vi "Read UI Configuration.vi"(8 "error in":errorcluster, 11 "Bus in":refnum<class "Bus.lvclass">) -> (0 "error out":errorcluster, 2 "UI Configuration":T1, 3 "Bus out":refnum<class "Bus.lvclass">)   [LabVIEW 2014, in "Bus.lvclass"]
uses:
  Bus.lvclass
  UI Configuration.ctl
  Bus Configuration/SPI Configuration.ctl
  Bus.lvclass/Bus.ctl
  Bus Configuration/Bus Configuration.lvclass/Bus Configuration.ctl
  <vilib>/NI/Configuration Framework/serializable configuration/NISE_CEF_serializable configuration.lvclass
  Bus Configuration/Bus Configuration.lvclass
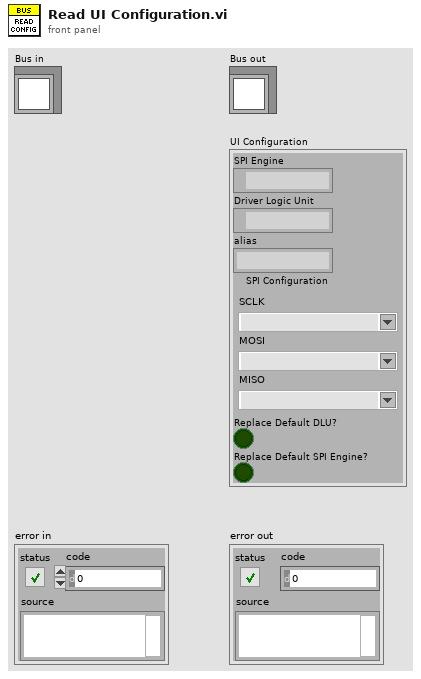
[diagram p1: front panel]
types:
  T1 = typedef "Bus.lvclass/UI Configuration.ctl" = cluster{"SPI Engine":path, "Driver Logic Unit":path, "alias":string, "SPI Configuration":T2, "Replace Default DLU?":bool, "Replace Default SPI Engine?":bool}
  T2 = typedef "Bus Configuration.lvclass/SPI Configuration.ctl" = cluster{"SCLK":string, "MOSI":string, "MISO":string}
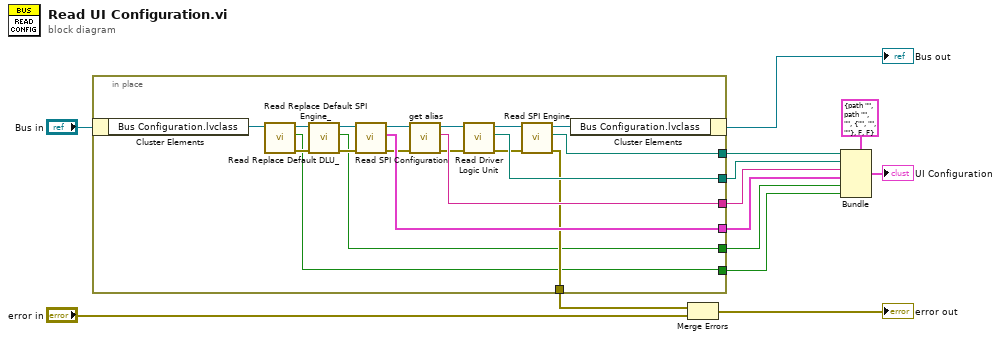
[diagram p0: block diagram]
diagram:
  n1 = in-place {
    in-place-border: [w28] -> w8
    in-place-border: [w27] -> w7
    in-place-border: [w26] -> w6
    in-place-border: [w25] -> w5
    in-place-border: [w21] -> w11
    in-place-border: [w18] -> w4
    in-place-border: [w14] -> w3
    n2 = in-place-cluster #1("Bus in") -> ("Bus Configuration.lvclass"=w17:refnum<class "Bus Configuration.lvclass">)
    n3 = call "Read Replace Default SPI Engine_.vi"("Bus Configuration in"=w17) -> ("error out"=w15:errorcluster, "Replace Default SPI Engine?"=w14:bool, "Bus Configuration out"=w16:refnum<class "Bus Configuration.lvclass">)  [unwired: 8 in]
    n4 = call "Read Replace Default DLU_.vi"("error in (no error)"=w15, "Bus Configuration in"=w16) -> ("error out"=w19:errorcluster, "Replace Default DLU?"=w18:bool, "Bus Configuration out"=w20:refnum<class "Bus Configuration.lvclass">)  [unwired: 7 in]
    n5 = call "Read SPI Configuration.vi"("error in (no error)"=w19, "Bus Configuration in"=w20) -> ("error out"=w24:errorcluster, "SPI Configuration"=w25:T2, "Bus Configuration out"=w32:refnum<class "Bus Configuration.lvclass">)  [unwired: 7 in]
    n6 = call <vilib>:"get alias.vi"("error in"=w24, "configuration in"=w32) -> ("error out"=w23:errorcluster, "alias"=w26:string, "configuration out"=w31:refnum<class "Bus Configuration.lvclass">)  [unwired: 7 in]
    n7 = call "Read Driver Logic Unit.vi"("error in (no error)"=w23, "Bus Configuration in"=w31) -> ("error out"=w22:errorcluster, "Driver Logic Unit"=w27:path, "Bus Configuration out"=w30:refnum<class "Bus Configuration.lvclass">)  [unwired: 7 in]
    n8 = call "Read SPI Engine.vi"("error in (no error)"=w22, "Bus Configuration in"=w30) -> ("error out"=w21:errorcluster, "SPI Engine"=w28:path, "Bus Configuration out"=w29:refnum<class "Bus Configuration.lvclass">)  [unwired: 7 in]
    n9 = in-place-cluster #1("Bus Configuration.lvclass"=w29) -> (→"Bus out":refnum<class "Bus.lvclass">)
  }
  n10 = Merge Errors(w11, "error in") -> (→"error out":errorcluster)
  n11 = Bundle(cluster=T1 {"SPI Engine"=path "", "Driver Logic Unit"=path "", "alias"="", "SPI Configuration"={"SCLK"="", "MOSI"="", "MISO"=""}, "Replace Default DLU?"=FALSE, "Replace Default SPI Engine?"=FALSE} ("UI Configuration"), "SPI Engine"=w8, "Driver Logic Unit"=w7, "alias"=w6, "SPI Configuration"=w5, "Replace Default DLU?"=w4, "Replace Default SPI Engine?"=w3) -> (→"UI Configuration":T1)
